vi "UpdateControl.vi"(8 "error in (no error)":errorcluster, 11 "Experiment in":refnum<class "Experiment.lvclass">) -> (0 "error out":errorcluster, 3 "Experiment out":refnum<class "Experiment.lvclass">)   [LabVIEW 2014, in "Experiment.lvclass"]
uses:
  Experiment.lvclass
  Experiment.lvclass/Experiment.ctl
  Database/Database.lvclass
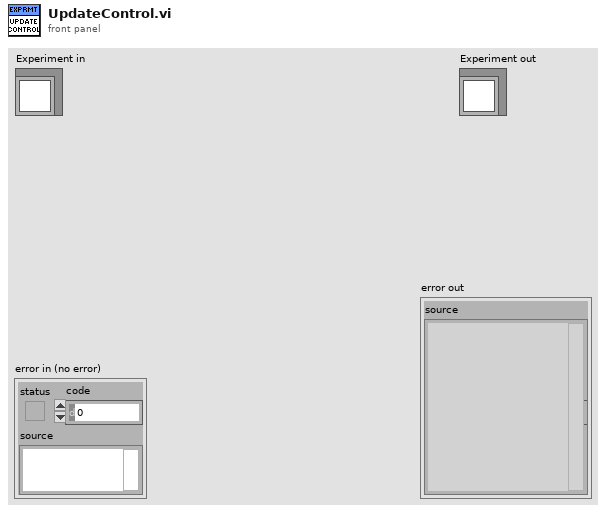
[diagram p1: front panel]
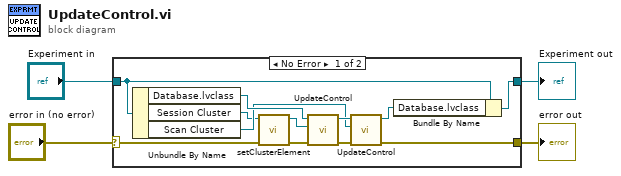
[diagram p0: block diagram]
diagram:
  n1 = case shown="No Error" "error in (no error)" {
    selector: "error in (no error)" -> [w6 w18]
    tunnel: [w10 w18] -> w4
    tunnel: [w14 w17] -> w2
    tunnel: "Experiment in" -> [w15 w17]
    frame No Error {
      n2 = Unbundle By Name(w15) -> ("Database.lvclass"=w16:refnum<class "Database.lvclass">, "Session Cluster"=w8:refnum<vi>, "Scan Cluster"=w9:refnum<vi>)
      n3 = call "setClusterElement.vi"("error in (no error)"=w6, "reference"=w8) -> ("error out"=w5:errorcluster, "reference 2"=w7:refnum<vi>)  [unwired: 8 in]
      n4 = call-dynamic "UpdateControl.vi"("error in (no error)"=w5, "Clust Refnum"=w7, "Database in"=w16) -> ("error out"=w11:errorcluster, "Database out"=w13:refnum<class "Database.lvclass">)  [unwired: 7 in]
      n5 = call-dynamic "UpdateControl.vi"("error in (no error)"=w11, "Clust Refnum"=w9, "Database in"=w13) -> ("error out"=w10:errorcluster, "Database out"=w12:refnum<class "Database.lvclass">)  [unwired: 7 in]
      n6 = Bundle By Name(cluster=w15, "Database.lvclass"=w12) -> (w14:refnum<class "Experiment.lvclass">)
    }
    frame Error {
    }
  }
  "error out" <- w4
  "Experiment out" <- w2
